vi "Read Calibration.vi"(8 "error in (no error)":errorcluster, 11 "Analyze Parameter Calibration in":refnum<class "Analyze Parameter Calibration.lvclass">) -> (0 "error out":errorcluster, 2 "Calibration":dbl[unit], 3 "Analyze Parameter Calibration out":refnum<class "Analyze Parameter Calibration.lvclass">)   [LabVIEW 2014, in "Analyze Parameter Calibration.lvclass"]
uses:
  Analyze Parameter Calibration.lvclass
  Analyze Parameter Calibration.lvclass/Analyze Parameter Calibration.ctl
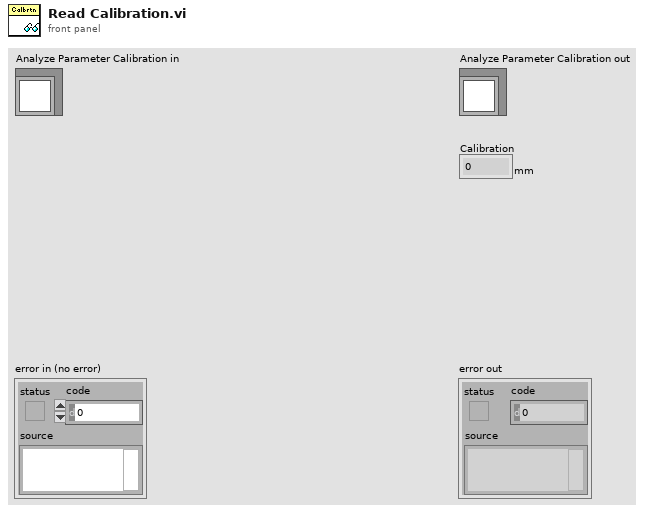
[diagram p1: front panel]
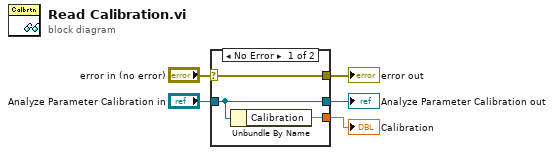
[diagram p0: block diagram]
diagram:
  n1 = case shown="No Error" "error in (no error)" {
    selector: "error in (no error)" -> [w8 w9]
    tunnel: [w8 w9] -> w4
    tunnel: [w7 w10] -> w2
    tunnel: "Analyze Parameter Calibration in" -> [w7 w10]
    tunnel: [w6 _] -> w1
    frame No Error {
      n2 = Unbundle By Name(w7) -> ("Calibration"=w6:dbl[unit])
    }
    frame Error {
    }
  }
  "error out" <- w4
  "Analyze Parameter Calibration out" <- w2
  "Calibration" <- w1
